vi "Poly Set Map Details.vi"(10 "Poly VI Name":string, 11 "Poly Set Map in":T2) -> (3 "Poly Details":T1[](array[typedef]))   [LabVIEW 2020]
uses:
  _td_map_PolyInstanceInfo.ctl
  _td_cluster_InstanceInfo.ctl
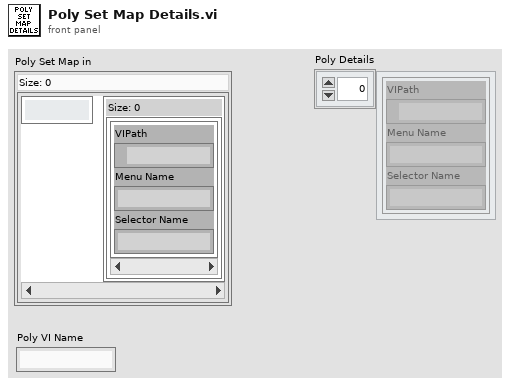
[diagram p1: front panel]
types:
  T1 = typedef "_td_cluster_InstanceInfo.ctl" = cluster{"VIPath":path, "Menu Name":string, "Selector Name":string}
  T2 = typedef "_td_map_PolyInstanceInfo.ctl" = map{string, set{T1}}
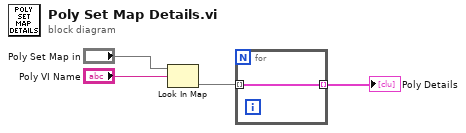
[diagram p0: block diagram]
diagram:
  n1 = Look In Map(map="Poly Set Map in", key="Poly VI Name") -> (value=w2:set{T1})  [unwired: 1 in, 1 out]
  n2 = for {
    tunnel: [w5] -> w1 mode=indexing
    tunnel: w2 -> [w5] mode=indexing
  }
  "Poly Details" <- w1
